vi "Untitled3.vi"() -> ()   [LabVIEW 2024]
uses:
  HAL/HAL/Devices/CAN Interfaces/PCAN/PCAN.lvclass
  HAL/HAL/Configurations/CFG Base/CFG Base.lvclass
  TickCount/TickCount.dll
  CANopen Master.lvlib
  HAL/HAL/Time Stamp/Time Stamp.lvclass
panel:
  out ".NET":dbl format="%#_g s"
  out "tick countPC DLL":dbl
  out "tick count64 DLL":dbl
  out "tick count DLL":dbl
  out "tick count":dbl
  out "High Res":dbl
  in  "Stop":bool
  out "error out":errorcluster
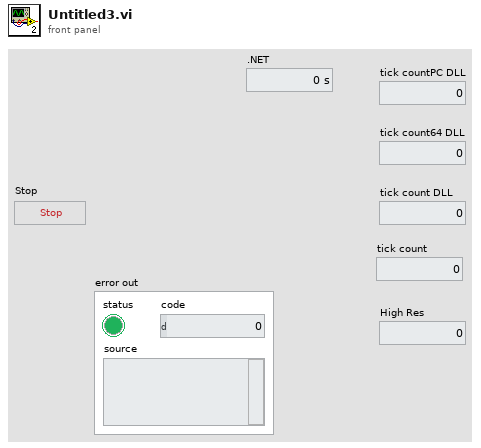
[diagram p1: front panel]
types:
  T1 = cluster{"ID":u32, "MSG type":u8, "DLC":u8, "Time Stamp":refnum<class "Time Stamp.lvclass">, "DATA":u8[]}
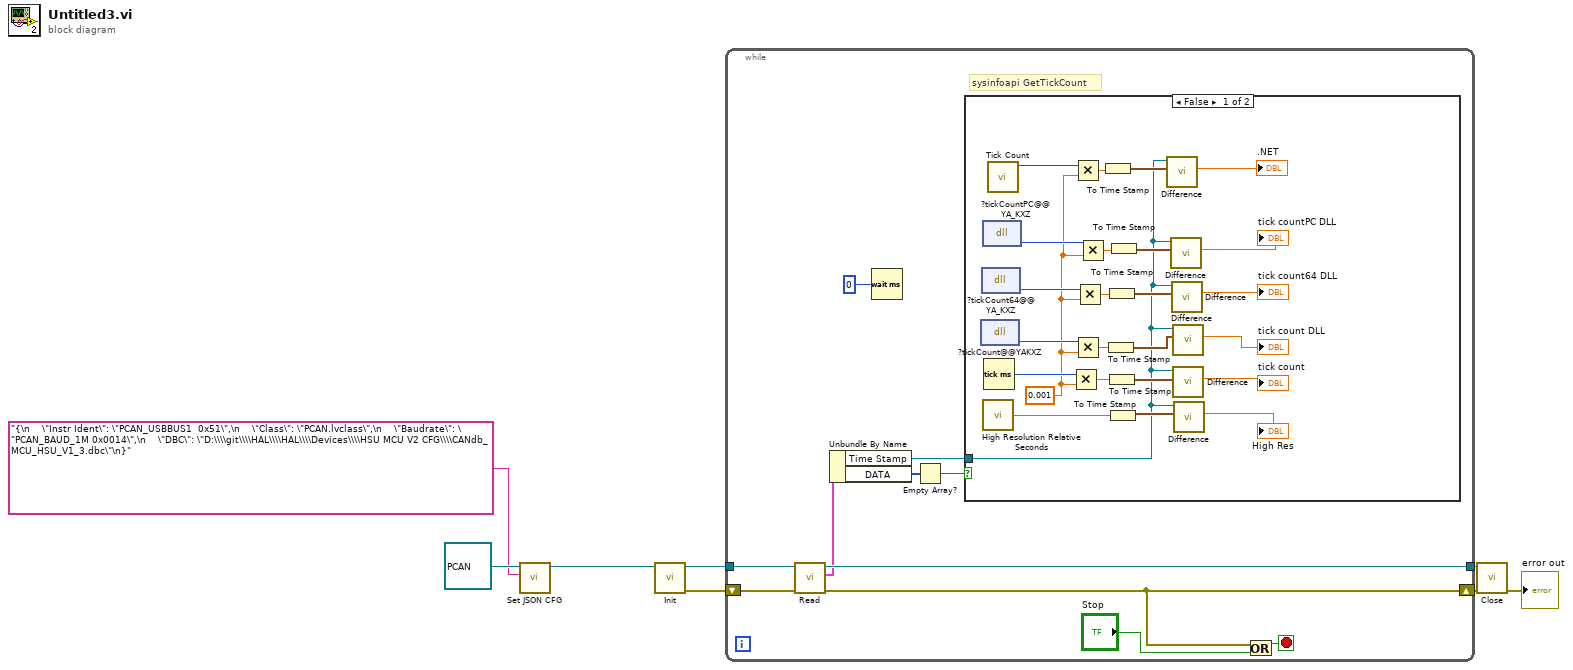
[diagram p0: block diagram]
diagram:
  n1 = call "Set JSON CFG.vi"("<JSON>CFG"="{\n    \"Instr Ident\": \"PCAN_USBBUS1  0x51\",\n    \"Class\": \"PCAN.lvclass\",\n    \"Baudrate\": \"PCAN_BAUD_1M 0x0014\",\n    \"DBC\": \"D:\\\\git\\\\HAL\\\\HAL\\\\Devices\\\\HSU MCU V2 CFG\\\\CANdb_MCU_HSU_V1_3.dbc\"\n}", "CFG Base in"=refnum<class "PCAN.lvclass"> refnum ("PCAN.lvclass")) -> ("CFG Base out"=w7:refnum<class "CFG Base.lvclass">)  [unwired: 9 in]
  n2 = call-dynamic "Init.vi"("PCAN in"=w7) -> ("error out"=w5:errorcluster, "PCAN out"=w4:refnum<class "PCAN.lvclass">)  [unwired: 9 in]
  n3 = while {
    tunnel: w4 -> [w18]
    shift-right: [w11] -> w3
    shift-left: w5 -> [w19]
    tunnel: [w16] -> w1
    stop <- w10 stop-if-true
    # "sysinfoapi GetTickCount"
    n4 = call-dynamic "Read.vi"("error in"=w19, "PCAN in"=w18) -> ("error out"=w11:errorcluster, "CAN Message"=w15:T1, "PCAN out"=w16:refnum<class "PCAN.lvclass">)  [unwired: 7 in]
    n5 = Unbundle By Name(w15) -> ("Time Stamp"=w14:refnum<class "Time Stamp.lvclass">, "DATA"=w13:u8[])
    n6 = Wait (ms)(milliseconds to wait=u32 0) -> ()  [unwired: 1 out]
    n7 = Empty Array?(array=w13) -> (empty?=w12:bool)
    n8 = case shown="False" w12 {
      tunnel: w14 -> [w23 _]
      frame False {
        w21 = 0.001
        n9 = dll-call lib="D:/git/CANopen-XNET/TickCount/TickCount.dll" fn="?tickCount@@YAKXZ" label="tickCount"() -> ("ticks"=w41:u32)  [unwired: 3 in, 2 out]
        n10 = dll-call lib="D:/git/CANopen-XNET/TickCount/TickCount.dll" fn="?tickCount64@@YA_KXZ" label="tickCount64"() -> ("ticks"=w39:u64)  [unwired: 3 in, 2 out]
        n11 = dll-call lib="D:/git/CANopen-XNET/TickCount/TickCount.dll" fn="?tickCountPC@@YA_KXZ" label="tickCountPC"() -> ("ticks"=w29:u64)  [unwired: 3 in, 2 out]
        n12 = call <vilib>:"High Resolution Relative Seconds.vi"() -> ("relative seconds"=w43:dbl)
        n13 = Tick Count (ms)() -> (millisecond timer value=w44:u32)
        n14 = call "Tick Count.vi"() -> ("Ticks"=w20:u64)  [unwired: 10 in, 1 out]
        n15 = Multiply(x=w44, y=w21) -> (x*y=w42:dbl)
        n16 = Multiply(x=w20, y=w21) -> (x*y=w25:dbl)
        n17 = Multiply(x=w41, y=w21) -> (x*y=w40:dbl)
        n18 = Multiply(x=w39, y=w21) -> (x*y=w30:dbl)
        n19 = Multiply(x=w29, y=w21) -> (x*y=w28:dbl)
        n20 = To Time Stamp(1:w25) -> (0:w24:timestamp)
        n21 = To Time Stamp(1:w40) -> (0:w37:timestamp)
        n22 = To Time Stamp(1:w30) -> (0:w38:timestamp)
        n23 = To Time Stamp(1:w42) -> (0:w36:timestamp)
        n24 = To Time Stamp(1:w43) -> (0:w35:timestamp)
        n25 = To Time Stamp(1:w28) -> (0:w27:timestamp)
        n26 = call "Difference.vi"("Time"=w24, "Time Stamp in"=w23) -> ("Difference"=→".NET":dbl)  [unwired: 7 in, 2 out]
        n27 = call "Difference.vi"("Time"=w27, "Time Stamp in"=w23) -> ("Difference"=→"tick countPC DLL":dbl)  [unwired: 7 in, 2 out]
        n28 = call "Difference.vi"("Time"=w38, "Time Stamp in"=w23) -> ("Difference"=→"tick count64 DLL":dbl)  [unwired: 7 in, 2 out]
        n29 = call "Difference.vi"("Time"=w37, "Time Stamp in"=w23) -> ("Difference"=→"tick count DLL":dbl)  [unwired: 7 in, 2 out]
        n30 = call "Difference.vi"("Time"=w36, "Time Stamp in"=w23) -> ("Difference"=→"tick count":dbl)  [unwired: 7 in, 2 out]
        n31 = call "Difference.vi"("Time"=w35, "Time Stamp in"=w23) -> ("Difference"=→"High Res":dbl)  [unwired: 7 in, 2 out]
      }
      frame True {
      }
    }
    n32 = Or(x=w11, y="Stop") -> (x .or. y?=w10:bool)
  }
  n33 = call-dynamic "Close.vi"("error in"=w3, "PCAN in"=w1) -> ("error out"=→"error out":errorcluster)  [unwired: 8 in, 1 out]
